vi "PPMS.Chamber Status Ring to String.vi"(1 "Chamber Status":T1 items=["ChamberUnknown"=0, "PurgedAndSealed"=1, "VentedAndSealed"=2, "Sealed"=3, "Purging"=4, "Venting"=5, "PreHiVac"=6, "HighVac"=7, "PumpContinuous"=8, "VentContinuous"=9, "ChamberFailure"=15]) -> (0 "Status String":string)   [LabVIEW 2019, in "instrument.PPMS.lvclass"]
uses:
  instrument.PPMS.lvclass
  Typedefs/PPMS.Chamber Status--ring.ctl
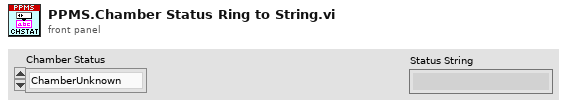
[diagram p1: front panel]
types:
  T1 = typedef "instrument.PPMS.lvclass/PPMS.Chamber Status--ring.ctl" = i32
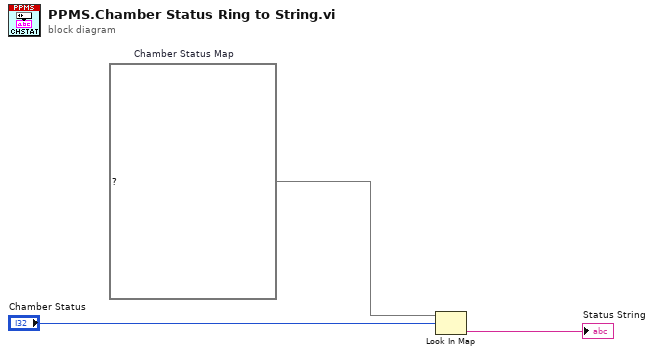
[diagram p0: block diagram]
diagram:
  w1 = map{i32, string} {0="ChamberUnknown", 1="PurgedAndSealed", 2="VentedAndSealed", 3="Sealed", 4="Purging", 5="Venting", 6="PreHiVac", 7="HighVac", 8="PumpContinuous", 9="VentContinuous", 15="ChamberFailure"}  # Chamber Status Map
  n1 = Look In Map(map=w1, key="Chamber Status") -> (value=→"Status String":string)  [unwired: 1 in, 1 out]
